vi "button actuation counter.vi"(11 "button pressed":bool) -> (3 "counter":i32)   [LabVIEW 2016]
panel:
  # "RETORNA O NÚMERO DE VEZES QUE A ENTRADA\nMUDA DE FALSE PARA TRUE."
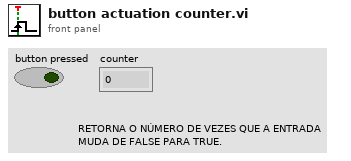
[diagram p1: front panel]
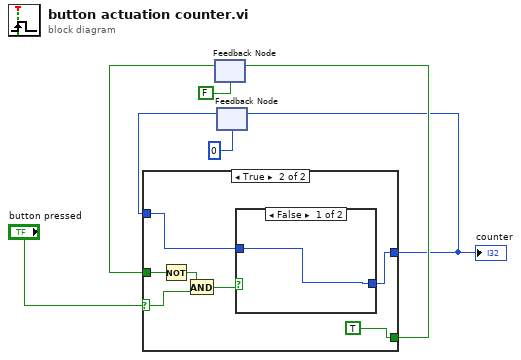
[diagram p0: block diagram]
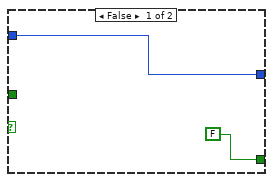
[diagram p2: hidden frame]
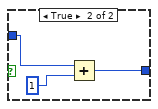
[diagram p3: hidden frame]
diagram:
  n1 = feedback #1(FALSE) -> (w6:bool)
  n2 = feedback #2(0 ("Numeric 2")) -> (w3:i32)
  n3 = case shown="True" "button pressed" {
    selector: "button pressed" -> [_ w11]
    tunnel: w3 -> [w9 w14]
    tunnel: [w9 w13] -> w2
    tunnel: w6 -> [_ w12]
    tunnel: [FALSE TRUE] -> w7
    frame False {
    }
    frame True {
      n4 = Not(x=w12) -> (.not. x?=w15:bool)
      n5 = And(x=w15, y=w11) -> (x .and. y?=w16:bool)
      n6 = case shown="False" w16 {
        tunnel: w14 -> [w17 w19]
        tunnel: [w17 w18] -> w13
        frame False {
        }
        frame True {
          n7 = Add(x=w19, y=1) -> (x+y=w18:i32)
        }
      }
    }
  }
  "counter" <- w2
  n8 = feedback-in #1(w7) -> ()
  n9 = feedback-in #2(w2) -> ()
